vi "servosistema.vi"() -> ()   [LabVIEW 2012]
uses:
  Instance           1 21Saved   Regulador PID .vi
panel:
  in  "k2o":dbl(slide) scale=-50.0..50.0
  in  "k1o":dbl(slide) scale=-50.0..50.0
  out "Control":dbl(graph)
  in  "k1":dbl(slide) scale=-50.0..50.0
  in  "k2":dbl(slide) scale=-50.0..50.0
  in  "ki":dbl(slide) scale=-50.0..50.0
  in  "salida":bool
  out "Respuesta":dynamicdata(graph)
  out "Error":dbl(graph)
  in  "Tiempo de Muestreo":dbl
  in  "stop":bool
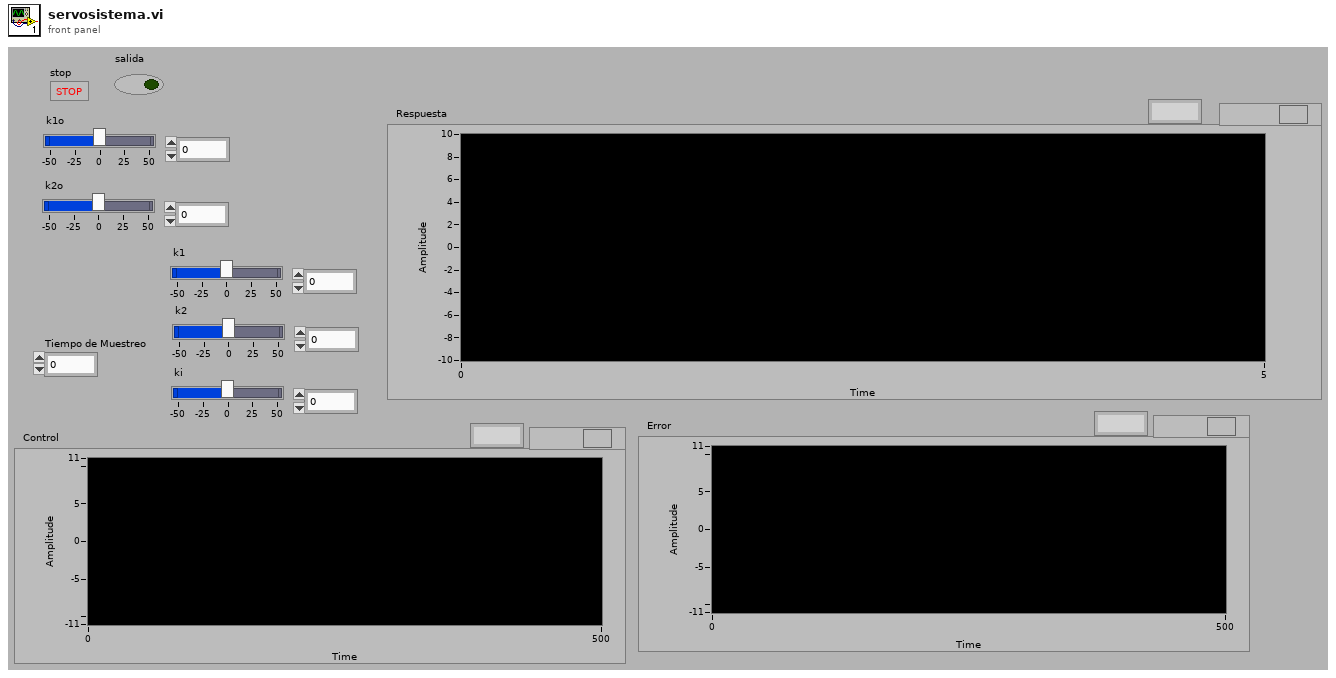
[diagram p1: front panel]
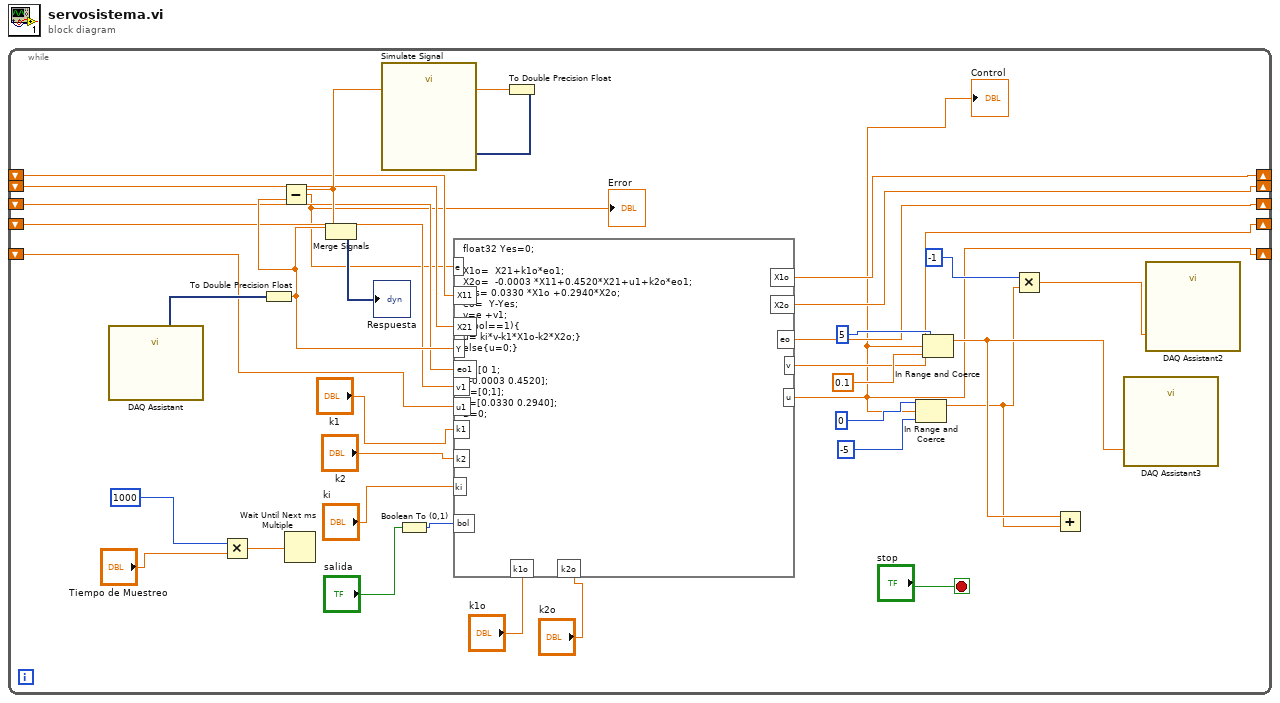
[diagram p0: block diagram]
diagram:
  n1 = while {
    shift-right: [w17] -> _
    shift-left: _ -> [w15]
    shift-right: [w16] -> _
    shift-left: _ -> [w14]
    shift-right: [w10] -> _
    shift-left: _ -> [w9]
    shift-right: [w8] -> _
    shift-left: _ -> [w7]
    shift-right: [w4] -> _
    shift-left: _ -> [w5]
    stop <- "stop" stop-if-true
    n2 = call "DAQ Assistant"() -> ("data"=w29:dynamicdata)  [unwired: 17 in, 2 out]
    n3 = Multiply(x=1000, y="Tiempo de Muestreo") -> (x*y=w33:dbl)
    n4 = To Double Precision Float(number=w29) -> (double precision float=w11:dbl)
    n5 = Wait Until Next ms Multiple(millisecond multiple=w33) -> ()  [unwired: 1 out]
    n6 = call "Simulate Signal"() -> ("Square"=w22:dynamicdata)  [unwired: 14 in, 1 out]
    n7 = Boolean To (0,1)(Boolean="salida") -> (0, 1=w20:i16)
    n8 = To Double Precision Float(number=w22) -> (double precision float=w18:dbl)
    n9 = Subtract(x=w18, y=w11) -> (x-y=w3:dbl)
    "Error" <- w3
    n10 = Merge Signals(w11, w18) -> (→"Respuesta":dynamicdata)
    n11 = formula code="float32 Yes=0;\n\nX1o=  X21+k1o*eo1;\nX2o=  -0.0003 *X11+0.4520*X21+u1+k2o*eo1;\nYes= 0.0330 *X1o +0.2940*X2o;\neo=  Y-Yes;\nv=e +v1;\nif(bol==1){\nu= ki*v-k1*X1o-k2*X2o;}\nelse{u=0;}\n\nG=[0 1;\n  -0.0003 0.4520];\nH=[0;1];\nC=[0.0330 0.2940];\nD=0;"("k1"="k1", "k2"="k2", "bol"=w20, "e"=w3, "X11"=w15, "X21"=w14, "eo1"=w9, "u1"=w5, "Y"=w11, "v1"=w7, "ki"="ki", "k1o"="k1o", "k2o"="k2o") -> ("X1o"=w17:dbl, "X2o"=w16:dbl, "eo"=w10:dbl, "v"=w8:dbl, "u"=w4:dbl)
    "Control" <- w4
    n12 = In Range and Coerce(upper limit=0, x=w4, lower limit=-5) -> (coerced(x)=w24:dbl)  [unwired: 1 out]
    n13 = In Range and Coerce(upper limit=5, x=w4, lower limit=0.1) -> (coerced(x)=w25:dbl)  [unwired: 1 out]
    n14 = Multiply(x=-1, y=w24) -> (x*y=w26:dbl)
    n15 = Add(x=w25, y=w24) -> ()  [unwired: 1 out]
    n16 = call "DAQ Assistant3"("data"=w25) -> ()  [unwired: 17 in, 2 out]
    n17 = call "DAQ Assistant2"("data"=w26) -> ()  [unwired: 17 in, 2 out]
  }
